vi "FormatDMAelement_4_elements.vi"(8 "valid in":bool, 10 "factor":u16, 11 "Array":T1=[0.0, 0.0, 0.0, 0.0, 0.0, 0.0, 0.0, 0.0]) -> (0 "valid out":bool, 3 "Values":u64[](array[numeric]))   [LabVIEW 2025]
uses:
  Array-18bit-8element.ctl
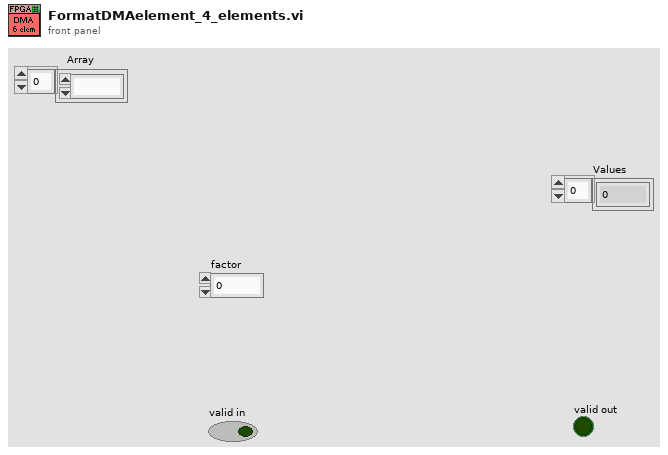
[diagram p1: front panel]
types:
  T1 = typedef "Array-18bit-8element.ctl" = fxp<+/-,18,1>[]
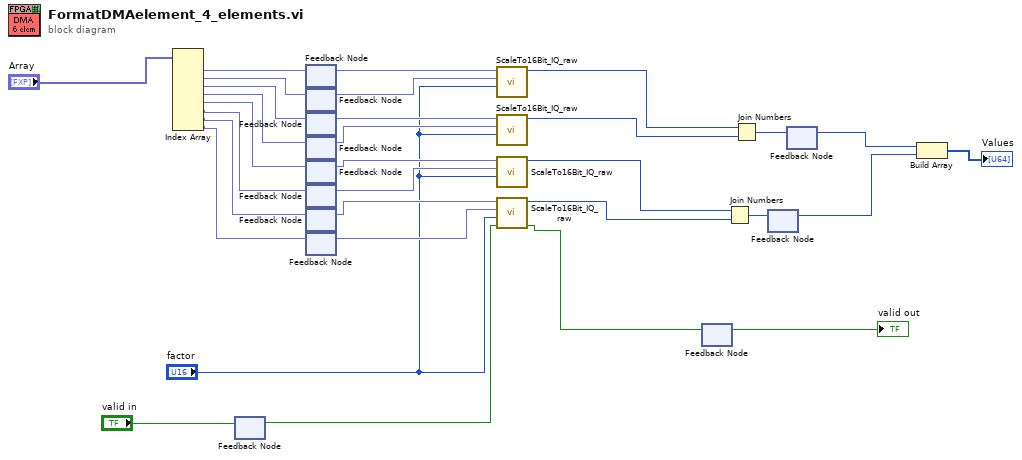
[diagram p0: block diagram]
diagram:
  n1 = Index Array(array="Array") -> (element #1=w31:fxp<+/-,18,1>, element #2=w30:fxp<+/-,18,1>, element #3=w29:fxp<+/-,18,1>, element #4=w28:fxp<+/-,18,1>, element #5=w16:fxp<+/-,18,1>, element #6=w15:fxp<+/-,18,1>, element #7=w14:fxp<+/-,18,1>, element #8=w13:fxp<+/-,18,1>)  [unwired: 8 in]
  n2 = feedback #1() -> (w5:bool)  [unwired: 1 in]
  n3 = feedback-in #1("valid in") -> ()
  n4 = feedback #2() -> (w21:fxp<+/-,18,1>)  [unwired: 1 in]
  n5 = feedback-in #2(w31) -> ()
  n6 = feedback #3() -> (w17:fxp<+/-,18,1>)  [unwired: 1 in]
  n7 = feedback-in #3(w30) -> ()
  n8 = feedback #4() -> (w12:fxp<+/-,18,1>)  [unwired: 1 in]
  n9 = feedback-in #4(w29) -> ()
  n10 = feedback #5() -> (w11:fxp<+/-,18,1>)  [unwired: 1 in]
  n11 = feedback-in #5(w28) -> ()
  n12 = feedback #6() -> (w10:fxp<+/-,18,1>)  [unwired: 1 in]
  n13 = feedback-in #6(w16) -> ()
  n14 = feedback #7() -> (w9:fxp<+/-,18,1>)  [unwired: 1 in]
  n15 = feedback-in #7(w15) -> ()
  n16 = feedback #8() -> (w8:fxp<+/-,18,1>)  [unwired: 1 in]
  n17 = feedback-in #8(w14) -> ()
  n18 = feedback #9() -> (w7:fxp<+/-,18,1>)  [unwired: 1 in]
  n19 = feedback-in #9(w13) -> ()
  n20 = call "ScaleTo16Bit_IQ_raw.vi"("factor"="factor", "Q"=w17, "I"=w21) -> ("32bit integer"=w20:u32)  [unwired: 7 in, 1 out]
  n21 = call "ScaleTo16Bit_IQ_raw.vi"("factor"="factor", "Q"=w11, "I"=w12) -> ("32bit integer"=w1:u32)  [unwired: 7 in, 1 out]
  n22 = call "ScaleTo16Bit_IQ_raw.vi"("factor"="factor", "Q"=w9, "I"=w10) -> ("32bit integer"=w3:u32)  [unwired: 7 in, 1 out]
  n23 = call "ScaleTo16Bit_IQ_raw.vi"("valid in"=w5, "factor"="factor", "Q"=w7, "I"=w8) -> ("valid out"=w4:bool, "32bit integer"=w2:u32)  [unwired: 6 in]
  n24 = feedback #10() -> (→"valid out":bool)  [unwired: 1 in]
  n25 = feedback-in #10(w4) -> ()
  n26 = Join Numbers(hi=w3, lo=w2) -> ((hi.lo)=w26:u64)
  n27 = Join Numbers(hi=w20, lo=w1) -> ((hi.lo)=w27:u64)
  n28 = feedback #11() -> (w25:u64)  [unwired: 1 in]
  n29 = feedback-in #11(w26) -> ()
  n30 = feedback #12() -> (w24:u64)  [unwired: 1 in]
  n31 = feedback-in #12(w27) -> ()
  n32 = Build Array(w24, w25) -> (→"Values":u64[])
